vi "HFRR ADV v013 new software.vi"() -> ()   [LabVIEW 2025] (continued)
              n2046 = Add(x=w2266, y=0.0) -> (x+y=w2262:dbl)
            }
            n2047 = for {
              N: w2154 -> [_]
              tunnel: w2161 -> [w2209]
              tunnel: w2160 -> [w2208]
              tunnel: [w2198] -> w2114 mode=indexing
              tunnel: [w2197] -> w2107 mode=indexing
              tunnel: w2151 -> [_]
              tunnel: [w2186] -> w2112 mode=indexing
              tunnel: [w2191] -> w2109 mode=indexing
              tunnel: [w2187] -> w2099 mode=indexing
              tunnel: [w2182] -> w2074 mode=indexing
              tunnel: [w2178] -> w2055 mode=indexing
              tunnel: [w2173] -> w2015 mode=indexing
              (unwired) 1.0 ("x")
              (unwired) TRUE ("line mode (F)")
              n2048 = Read from Text File "Read File"(file (use dialog)=w2209, error in=w2208) -> (text=w2174:string)  [unwired: 2 in, 3 out]
              n2049 = local write "String 12"(w2174) -> ()
              n2050 = String Subset(string=w2174, offset (0)=85, length (rest)=9 ("length (rest)")) -> (substring=w2176:string)
              n2051 = String Subset(string=w2174, offset (0)=35, length (rest)=9 ("length (rest)")) -> (substring=w2199:string)
              n2052 = String Subset(string=w2174, offset (0)=55, length (rest)=9 ("length (rest)")) -> (substring=w2184:string)
              n2053 = String Subset(string=w2174, offset (0)=25, length (rest)=9 ("length (rest)")) -> (substring=w2180:string)
              n2054 = String Subset(string=w2174, offset (0)=45, length (rest)=9 ("length (rest)")) -> (substring=w2189:string)
              n2055 = String Subset(string=w2174, offset (0)=15, length (rest)=9 ("length (rest)")) -> (substring=w2205:string)
              n2056 = String Subset(string=w2174, offset (0)=0, length (rest)=14 ("length (rest)")) -> (substring=w2202:string)
              n2057 = String Subset(string=w2174, offset (0)=65, length (rest)=9 ("length (rest)")) -> (substring=w2192:string)
              n2058 = Fract/Exp String To Number(string=w2176) -> (number=w2173:dbl)  [unwired: 3 in, 1 out]
              n2059 = Fract/Exp String To Number(string=w2199) -> (number=w2197:dbl)  [unwired: 3 in, 1 out]
              n2060 = Fract/Exp String To Number(string=w2184) -> (number=w2182:dbl)  [unwired: 3 in, 1 out]
              n2061 = Fract/Exp String To Number(string=w2180) -> (number=w2178:dbl)  [unwired: 3 in, 1 out]
              n2062 = Fract/Exp String To Number(string=w2189) -> (number=w2187:dbl)  [unwired: 3 in, 1 out]
              n2063 = Fract/Exp String To Number(string=w2205) -> (number=w2186:dbl)  [unwired: 3 in, 1 out]
              n2064 = Fract/Exp String To Number(string=w2202) -> (number=w2198:dbl)  [unwired: 3 in, 1 out]
              n2065 = Fract/Exp String To Number(string=w2192) -> (number=w2195:dbl)  [unwired: 3 in, 1 out]
              n2066 = Add(x=w2195, y=0.0) -> (x+y=w2191:dbl)
            }
            n2067 = Delete From Array(array=w2057, index=0) -> (array with subset deleted=w2030:dbl[])  [unwired: 1 in, 1 out]
            n2068 = Delete From Array(array=w2120, index=0) -> (array with subset deleted=w2093:dbl[])  [unwired: 1 in, 1 out]
            n2069 = Delete From Array(array=w2100, index=0) -> (array with subset deleted=w2088:dbl[])  [unwired: 1 in, 1 out]
            n2070 = Delete From Array(array=w2118, index=0) -> (array with subset deleted=w2119:dbl[])  [unwired: 1 in, 1 out]
            n2071 = call-poly <vilib>:"Mean.vi"("X"=w2030) -> ("mean"=→"КОФ2 4":dbl)  [unwired: 1 out]
            n2072 = call-poly <vilib>:"Mean.vi"("X"=w2093) -> ("mean"=→"КОФ3":dbl)  [unwired: 1 out]
            n2073 = call-poly <vilib>:"Mean.vi"("X"=w2088) -> ("mean"=→"CP3":dbl)  [unwired: 1 out]
            n2074 = Delete From Array(array=w2082, index=0) -> (array with subset deleted=w2009:dbl[])  [unwired: 1 in, 1 out]
            n2075 = Delete From Array(array=w2021, index=0) -> (array with subset deleted=w2008:dbl[])  [unwired: 1 in, 1 out]
            n2076 = Delete From Array(array=w2061, index=0) -> (array with subset deleted=w2032:dbl[])  [unwired: 1 in, 1 out]
            n2077 = Delete From Array(array=w2139, index=0) -> (array with subset deleted=w2094:dbl[])  [unwired: 1 in, 1 out]
            n2078 = Delete From Array(array=w2105, index=0) -> (array with subset deleted=w2090:dbl[])  [unwired: 1 in, 1 out]
            "array w/ subset deleted" <- w2090
            n2079 = Delete From Array(array=w2136, index=0) -> (array with subset deleted=w2137:dbl[])  [unwired: 1 in, 1 out]
            n2080 = call-poly <vilib>:"Mean.vi"("X"=w2032) -> ("mean"=→"КОФ2 2":dbl)  [unwired: 1 out]
            n2081 = call-poly <vilib>:"Mean.vi"("X"=w2094) -> ("mean"=→"КОФ1":dbl)  [unwired: 1 out]
            n2082 = Bundle "Bundle"(w2009, w2008) -> (w2014:cluster{dbl[], dbl[]})  [unwired: 1 in]
            n2083 = Bundle "Bundle"(w2009, w2137) -> (w2001:cluster{dbl[], dbl[]})  [unwired: 1 in]
            n2084 = Delete From Array(array=w2016, index=0) -> (array with subset deleted=w2004:dbl[])  [unwired: 1 in, 1 out]
            n2085 = Delete From Array(array=w2017, index=0) -> (array with subset deleted=w2006:dbl[])  [unwired: 1 in, 1 out]
            n2086 = Delete From Array(array=w2127, index=0) -> (array with subset deleted=w2128:dbl[])  [unwired: 1 in, 1 out]
            n2087 = Delete From Array(array=w2015, index=0) -> (array with subset deleted=w2002:dbl[])  [unwired: 1 in, 1 out]
            n2088 = Delete From Array(array=w2109, index=0) -> (array with subset deleted=w2110:dbl[])  [unwired: 1 in, 1 out]
            n2089 = Delete From Array(array=w2134, index=0) -> (array with subset deleted=w2040:dbl[])  [unwired: 1 in, 1 out]
            n2090 = Delete From Array(array=w2080, index=0) -> (array with subset deleted=w2036:dbl[])  [unwired: 1 in, 1 out]
            n2091 = Delete From Array(array=w2116, index=0) -> (array with subset deleted=w2038:dbl[])  [unwired: 1 in, 1 out]
            n2092 = Delete From Array(array=w2076, index=0) -> (array with subset deleted=w2034:dbl[])  [unwired: 1 in, 1 out]
            n2093 = Delete From Array(array=w2125, index=0) -> (array with subset deleted=w2039:dbl[])  [unwired: 1 in, 1 out]
            n2094 = Delete From Array(array=w2078, index=0) -> (array with subset deleted=w2035:dbl[])  [unwired: 1 in, 1 out]
            n2095 = Delete From Array(array=w2059, index=0) -> (array with subset deleted=w2031:dbl[])  [unwired: 1 in, 1 out]
            n2096 = Delete From Array(array=w2103, index=0) -> (array with subset deleted=w2089:dbl[])  [unwired: 1 in, 1 out]
            n2097 = Delete From Array(array=w2130, index=0) -> (array with subset deleted=w2091:dbl[])  [unwired: 1 in, 1 out]
            n2098 = Delete From Array(array=w2107, index=0) -> (array with subset deleted=w2037:dbl[])  [unwired: 1 in, 1 out]
            n2099 = Delete From Array(array=w2074, index=0) -> (array with subset deleted=w2033:dbl[])  [unwired: 1 in, 1 out]
            n2100 = Delete From Array(array=w2055, index=0) -> (array with subset deleted=w2029:dbl[])  [unwired: 1 in, 1 out]
            n2101 = Delete From Array(array=w2099, index=0) -> (array with subset deleted=w2087:dbl[])  [unwired: 1 in, 1 out]
            n2102 = Delete From Array(array=w2112, index=0) -> (array with subset deleted=w2092:dbl[])  [unwired: 1 in, 1 out]
            n2103 = Delete From Array(array=w2122, index=0) -> (array with subset deleted=w2005:dbl[])  [unwired: 1 in, 1 out]
            n2104 = Delete From Array(array=w2132, index=0) -> (array with subset deleted=w2007:dbl[])  [unwired: 1 in, 1 out]
            n2105 = Delete From Array(array=w2114, index=0) -> (array with subset deleted=w2003:dbl[])  [unwired: 1 in, 1 out]
            n2106 = Bundle "Bundle"(w2009, w2040) -> (w2027:cluster{dbl[], dbl[]})  [unwired: 1 in]
            n2107 = Bundle "Bundle"(w2009, w2094) -> (w2028:cluster{dbl[], dbl[]})  [unwired: 1 in]
            n2108 = Bundle "Bundle"(w2040, w2036) -> (w2042:cluster{dbl[], dbl[]})  [unwired: 1 in]
            n2109 = Bundle "Bundle"(w2005, w2004) -> (w2012:cluster{dbl[], dbl[]})  [unwired: 1 in]
            n2110 = Bundle "Bundle"(w2038, w2034) -> (w2044:cluster{dbl[], dbl[]})  [unwired: 1 in]
            n2111 = Bundle "Bundle"(w2005, w2038) -> (w2148:cluster{dbl[], dbl[]})  [unwired: 1 in]
            n2112 = Bundle "Bundle"(w2005, w2034) -> (w2072:cluster{dbl[], dbl[]})  [unwired: 1 in]
            n2113 = Bundle "Bundle"(w2005, w2093) -> (w2158:cluster{dbl[], dbl[]})  [unwired: 1 in]
            n2114 = Bundle "Bundle"(w2005, w2088) -> (w2096:cluster{dbl[], dbl[]})  [unwired: 1 in]
            n2115 = Bundle "Bundle"(w2005, w2119) -> (w2143:cluster{dbl[], dbl[]})  [unwired: 1 in]
            n2116 = Bundle "Bundle"(w2039, w2035) -> (w2043:cluster{dbl[], dbl[]})  [unwired: 1 in]
            n2117 = Bundle "Bundle"(w2007, w2006) -> (w2013:cluster{dbl[], dbl[]})  [unwired: 1 in]
            n2118 = Bundle "Bundle"(w2007, w2039) -> (w2150:cluster{dbl[], dbl[]})  [unwired: 1 in]
            n2119 = Bundle "Bundle"(w2007, w2035) -> (w2073:cluster{dbl[], dbl[]})  [unwired: 1 in]
            n2120 = Bundle "Bundle"(w2007, w2089) -> (w2097:cluster{dbl[], dbl[]})  [unwired: 1 in]
            n2121 = Bundle "Bundle"(w2007, w2091) -> (w2159:cluster{dbl[], dbl[]})  [unwired: 1 in]
            n2122 = Bundle "Bundle"(w2007, w2128) -> (w2141:cluster{dbl[], dbl[]})  [unwired: 1 in]
            n2123 = Bundle "Bundle"(w2037, w2033) -> (w2045:cluster{dbl[], dbl[]})  [unwired: 1 in]
            n2124 = Bundle "Bundle"(w2003, w2002) -> (w2011:cluster{dbl[], dbl[]})  [unwired: 1 in]
            n2125 = Bundle "Bundle"(w2003, w2037) -> (w2149:cluster{dbl[], dbl[]})  [unwired: 1 in]
            n2126 = Bundle "Bundle"(w2003, w2033) -> (w2071:cluster{dbl[], dbl[]})  [unwired: 1 in]
            n2127 = Bundle "Bundle"(w2003, w2087) -> (w2095:cluster{dbl[], dbl[]})  [unwired: 1 in]
            n2128 = Bundle "Bundle"(w2003, w2092) -> (w2157:cluster{dbl[], dbl[]})  [unwired: 1 in]
            n2129 = Bundle "Bundle"(w2003, w2110) -> (w2142:cluster{dbl[], dbl[]})  [unwired: 1 in]
            n2130 = call-poly <vilib>:"Mean.vi"("X"=w2090) -> ("mean"=→"CP1":dbl)  [unwired: 1 out]
            n2131 = call-poly <vilib>:"Mean.vi"("X"=w2031) -> ("mean"=→"КОФ2 3":dbl)  [unwired: 1 out]
            n2132 = call-poly <vilib>:"Mean.vi"("X"=w2089) -> ("mean"=→"CP2":dbl)  [unwired: 1 out]
            n2133 = call-poly <vilib>:"Mean.vi"("X"=w2091) -> ("mean"=→"КОФ2":dbl)  [unwired: 1 out]
            n2134 = call-poly <vilib>:"Mean.vi"("X"=w2029) -> ("mean"=→"КОФ2 5":dbl)  [unwired: 1 out]
            n2135 = call-poly <vilib>:"Mean.vi"("X"=w2087) -> ("mean"=→"CP4":dbl)  [unwired: 1 out]
            n2136 = call-poly <vilib>:"Mean.vi"("X"=w2092) -> ("mean"=→"КОФ4":dbl)  [unwired: 1 out]
            n2137 = Bundle "Bundle"(w2009, w2036) -> (w2000:cluster{dbl[], dbl[]})  [unwired: 1 in]
            n2138 = Bundle "Bundle"(w2009, w2090) -> (w2023:cluster{dbl[], dbl[]})  [unwired: 1 in]
            n2139 = Build Array "Build Array"(w2000, w2023) -> (w2026:cluster{dbl[], dbl[]}[])
            "XY Graph 17" <- w2026
            n2140 = Build Array "Build Array"(w2014, w2013, w2012, w2011) -> (→"Frequency ( Hz )":cluster{dbl[], dbl[]}[])
            n2141 = Build Array "Build Array"(w2042, w2043, w2044, w2045) -> (→"Air Temp ( °C ) vs Humidity ( % RH )":cluster{dbl[], dbl[]}[])
            n2142 = Build Array "Build Array"(w2027, w2150, w2148, w2149) -> (→"Air Temperature  ( °C )":cluster{dbl[], dbl[]}[])
            n2143 = Build Array "Build Array"(w2000, w2073, w2072, w2071) -> (→"Humidity ( %RH )":cluster{dbl[], dbl[]}[])
            n2144 = Build Array "Build Array"(w2028, w2159, w2158, w2157) -> (→"Coefficient Of Friction":cluster{dbl[], dbl[]}[])
            n2145 = Build Array "Build Array"(w2023, w2097, w2096, w2095) -> (→"Sample Temperature ( °C )":cluster{dbl[], dbl[]}[])
            n2146 = Build Array "Build Array"(w2001, w2141, w2143, w2142) -> (→"XY Graph 13":cluster{dbl[], dbl[]}[])
            n2147 = Bundle "Bundle"(w2009, w2032) -> (w2054:cluster{dbl[], dbl[]})  [unwired: 1 in]
            n2148 = Bundle "Bundle"(w2005, w2030) -> (w2052:cluster{dbl[], dbl[]})  [unwired: 1 in]
            n2149 = Bundle "Bundle"(w2007, w2031) -> (w2053:cluster{dbl[], dbl[]})  [unwired: 1 in]
            n2150 = Bundle "Bundle"(w2003, w2029) -> (w2051:cluster{dbl[], dbl[]})  [unwired: 1 in]
            n2151 = Build Array "Build Array"(w2054, w2053, w2052, w2051) -> (→"Stroke ( mm )":cluster{dbl[], dbl[]}[])
            n2152 = local write "XY Graph 16"(w2026) -> ()
          }
          frame #2 {
          }
          frame #3 {
            n2153 = local write "Numeric 8"(0 ("Numeric 8")) -> ()
            n2154 = local write "Numeric 11"(0 ("Numeric 11")) -> ()
            n2155 = local write "Numeric 12"(0 ("Numeric 12")) -> ()
            n2156 = local write "Numeric 13"(0 ("Numeric 13")) -> ()
            n2157 = property on="OPEN" class="Bool (strict)"("Visible"=TRUE) -> ()  [unwired: 2 in, 2 out]
            n2158 = local read "String Control 2"() -> (w2326:string)
            n2159 = local read "String Control 4"() -> (w2325:string)
            n2160 = local read "String Control 6"() -> (w2324:string)
            n2161 = local read "String Control 8"() -> (w2323:string)
            n2162 = Match Pattern(string=w2326, regular expression="Samples / cycle :- ") -> (after substring=w2340:string)  [unwired: 1 in, 3 out]
            n2163 = Match Pattern(string=w2326, regular expression="Frequency :- ") -> (after substring=w2359:string)  [unwired: 1 in, 3 out]
            n2164 = Match Pattern(string=w2325, regular expression="Samples / cycle :- ") -> (after substring=w2336:string)  [unwired: 1 in, 3 out]
            n2165 = Match Pattern(string=w2325, regular expression="Frequency :- ") -> (after substring=w2354:string)  [unwired: 1 in, 3 out]
            n2166 = Match Pattern(string=w2324, regular expression="Samples / cycle :- ") -> (after substring=w2332:string)  [unwired: 1 in, 3 out]
            n2167 = Match Pattern(string=w2324, regular expression="Frequency :- ") -> (after substring=w2349:string)  [unwired: 1 in, 3 out]
            n2168 = Match Pattern(string=w2323, regular expression="Samples / cycle :- ") -> (after substring=w2328:string)  [unwired: 1 in, 3 out]
            n2169 = Match Pattern(string=w2323, regular expression="Frequency :- ") -> (after substring=w2344:string)  [unwired: 1 in, 3 out]
            n2170 = String Subset(string=w2340, length (rest)=6 ("length (rest)")) -> (substring=w2342:string)  [unwired: 1 in]
            n2171 = String Subset(string=w2359, length (rest)=9 ("length (rest)")) -> (substring=w2361:string)  [unwired: 1 in]
            n2172 = String Subset(string=w2336, length (rest)=6 ("length (rest)")) -> (substring=w2338:string)  [unwired: 1 in]
            n2173 = String Subset(string=w2354, length (rest)=9 ("length (rest)")) -> (substring=w2356:string)  [unwired: 1 in]
            n2174 = String Subset(string=w2332, length (rest)=6 ("length (rest)")) -> (substring=w2334:string)  [unwired: 1 in]
            n2175 = String Subset(string=w2349, length (rest)=9 ("length (rest)")) -> (substring=w2351:string)  [unwired: 1 in]
            n2176 = String Subset(string=w2328, length (rest)=6 ("length (rest)")) -> (substring=w2330:string)  [unwired: 1 in]
            n2177 = String Subset(string=w2344, length (rest)=9 ("length (rest)")) -> (substring=w2346:string)  [unwired: 1 in]
            n2178 = Fract/Exp String To Number(string=w2342) -> (number=w2322:dbl)  [unwired: 3 in, 1 out]
            n2179 = Fract/Exp String To Number(string=w2361) -> (number=w2362:dbl)  [unwired: 3 in, 1 out]
            n2180 = Fract/Exp String To Number(string=w2338) -> (number=w2321:dbl)  [unwired: 3 in, 1 out]
            n2181 = Fract/Exp String To Number(string=w2356) -> (number=w2357:dbl)  [unwired: 3 in, 1 out]
            n2182 = Fract/Exp String To Number(string=w2334) -> (number=w2320:dbl)  [unwired: 3 in, 1 out]
            n2183 = Fract/Exp String To Number(string=w2351) -> (number=w2352:dbl)  [unwired: 3 in, 1 out]
            n2184 = Fract/Exp String To Number(string=w2330) -> (number=w2319:dbl)  [unwired: 3 in, 1 out]
            n2185 = Fract/Exp String To Number(string=w2346) -> (number=w2347:dbl)  [unwired: 3 in, 1 out]
            n2186 = local write "sample1"(w2322) -> ()
            n2187 = local write "freq1"(w2362) -> ()
            n2188 = local write "sample2"(w2321) -> ()
            n2189 = local write "freq2"(w2357) -> ()
            n2190 = local write "sample3"(w2320) -> ()
            n2191 = local write "freq3"(w2352) -> ()
            n2192 = local write "sample4"(w2319) -> ()
            n2193 = local write "freq 4"(w2347) -> ()
          }
        }
      }
    }
    n2194 = case shown="True" w1811 {
      selector: w1811 -> [_ w1939]
      frame False {
      }
      frame True {
        n2195 = Not(x=w1939) -> (.not. x?=w1935:bool)
        n2196 = local write "service 3"(w1935) -> ()
        n2197 = local write "OPEN 6"(w1935) -> ()
        n2198 = call <vilib>:"System Exec.vi"("wait until completion? (T)"=TRUE, "command line"="C:\\LAB-IQ\\Scar View.exe") -> ("error out"=→"error out 5":errorcluster)  [unwired: 6 in, 3 out]
      }
    }
    n2199 = case shown="\"Acquire\", Default" w1822 {
      frame "Acquire", Default {
        w2835 = 0.2 ("y")
        w2840 = 1.0 ("y")
        w2841 = 0.8 ("y")
        # "Elapsed time\ncof\nstroke\nAir temp\nTemp\nHumidity"
        n2200 = disable-structure shown="Disabled" {
          frame Disabled {
            n2201 = local read "Flag"() -> (w2858:dbl)
            n2202 = local read "RUN"() -> (w2855:bool)
            n2203 = Not(x=w2855) -> (.not. x?=w2854:bool)
            n2204 = Equal?(x=w2858, y=10.0) -> (x = y?=w2856:bool)
            n2205 = And(x=w2856, y=w2854) -> (x .and. y?=w2853:bool)
            n2206 = case shown="True" w2853 {
              frame False {
              }
              frame True {
                w2859 = FALSE ("Heater Button")
                n2207 = local write "Humidity"(w2859) -> ()
                n2208 = local write "Heater Button"(w2859) -> ()
              }
            }
          }
          frame Enabled {
          }
        }
        n2209 = disable-structure shown="Disabled" {
          frame Disabled {
            n2210 = case shown="True" {
              selector: _ -> [_ _]
              frame False {
              }
              frame True {
                w2950 = TRUE ("Heater")
                n2211 = local write "Humidity"(w2950) -> ()
                n2212 = local write "Heater Button"(w2950) -> ()
                n2213 = local read "TEST STANDARD"() -> (w2953:T3)
                n2214 = local read "TEST STANDARD"() -> (w2948:T3)
                n2215 = Equal?(x=w2953, y=enum16{"ASTM D6079", "ISO 12156", "Custom"}."ISO 12156" ("Test Standard")) -> (x = y?=w2951:bool)
                n2216 = Equal?(x=w2948, y=enum16{"ASTM D6079", "ISO 12156", "Custom"}."ASTM D6079" ("Test Standard")) -> (x = y?=w2947:bool)
                n2217 = case shown="True" w2951 {
                  frame False {
                  }
                  frame True {
                    n2218 = local write "Heater"(TRUE ("Heater")) -> ()
                    n2219 = local write "airtempflg"(FALSE ("airtempflg")) -> ()
                  }
                }
                n2220 = case shown="True" w2947 {
                  frame False {
                  }
                  frame True {
                    n2221 = local write "Heater"(FALSE ("Heater")) -> ()
                    n2222 = local write "airtempflg"(TRUE ("airtempflg")) -> ()
                  }
                }
              }
            }
          }
          frame Enabled {
          }
        }
        n2223 = stacked-sequence {
          frame #0 {
            n2224 = case shown="True" "RST FF" {
              frame False {
              }
              frame True {
                w3016 = 0.0 ("X Scale.Range:Maximum")
                n2225 = property on="Frictional Force ( N )" class="WFChart (strict)"("XScale.Maximum"=600.0 ("X Scale.Range:Maximum"), "XScale.Minimum"=w3016, "YScale.Maximum"=10.0 ("Y Scale.Range:Maximum"), "YScale.Minimum"=w3016) -> ()  [unwired: 2 in, 2 out]
              }
            }
          }
          frame #1 {
            n2226 = case shown="True" "RST TEMP" {
              frame False {
              }
              frame True {
                n2227 = property on="Temperature ( Deg C )" class="WFChart (strict)"("XScale.Minimum"=0.0 ("X Scale.Range:Minimum"), "XScale.Maximum"=600.0 ("X Scale.Range:Maximum"), "YScale.Minimum"=0.0 ("Y Scale.Range:Minimum"), "YScale.Maximum"=100.0 ("Y Scale.Range:Maximum")) -> ()  [unwired: 2 in, 2 out]
              }
            }
          }
          frame #2 {
            n2228 = case shown="True" "RSTCOF" {
              frame False {
              }
              frame True {
                n2229 = property on="Coefficient of Friction" class="WFChart (strict)"("XScale.Minimum"=0.0 ("X Scale.Range:Minimum"), "XScale.Maximum"=600.0 ("X Scale.Range:Maximum"), "YScale.Maximum"=1.0 ("X Scale.Range:Minimum"), "YScale.Minimum"=0.0 ("X Scale.Range:Minimum")) -> ()  [unwired: 2 in, 2 out]
              }
            }
          }
          frame #3 {
            n2230 = case shown="True" "RSTCOF 2" {
              frame False {
              }
              frame True {
                (unwired) 100.0 ("Y Scale.Range:Maximum")
                (unwired) 0.0 ("Y Scale.Range:Minimum")
                (unwired) 600.0 ("X Scale.Range:Maximum")
                (unwired) 0.0 ("X Scale.Range:Minimum")
              }
            }
          }
          frame #4 {
            n2231 = case shown="True" "RSTCOF 3" {
              frame False {
              }
              frame True {
                n2232 = property on="Electrical Contact Resistance ( % )" class="WFChart (strict)"("XScale.Minimum"=0.0 ("X Scale.Range:Minimum"), "XScale.Maximum"=600.0 ("X Scale.Range:Maximum"), "YScale.Minimum"=0.0 ("Y Scale.Range:Minimum"), "YScale.Maximum"=100.0 ("Y Scale.Range:Maximum")) -> ()  [unwired: 2 in, 2 out]
              }
            }
          }
        }
        n2233 = disable-structure shown="Disabled" {
          frame Disabled {
            n2234 = case shown="True" {
              selector: _ -> [_ _]
              frame False {
              }
              frame True {
                n2235 = local read "zflag 2"() -> (w2917:dbl)
                n2236 = local read "yflag"() -> (w2919:dbl)
                n2237 = Equal?(x=w2919, y=2.0 ("tflag")) -> (x = y?=w2921:bool)
                n2238 = Equal?(x=w2917, y=3.0 ("tflag")) -> (x = y?=w2920:bool)
                n2239 = And(x=w2921, y=w2920) -> (x .and. y?=w2915:bool)
                n2240 = case shown="True" w2915 {
                  frame False {
                  }
                  frame True {
                    w2946 = 0.0 ("zflag")
                    n2241 = local write "zflag"(w2946) -> ()
                    n2242 = local write "zflag 2"(w2946) -> ()
                    n2243 = Delete(path (use dialog)=path "C:/LAB-IQ-NXT/WO 2449 TT.sig" ("file path (dialog if empty)")) -> (deleted path=w2945:path)  [unwired: 4 in, 2 out]
                    n2244 = Delete(path (use dialog)=path "C:/LAB-IQ-NXT/WO 2449 TRH.sig" ("file path (dialog if empty)")) -> (deleted path=w2940:path)  [unwired: 4 in, 2 out]
                    n2245 = local read "SEN.RUN HRS"() -> (w2932:dbl)
                    n2246 = local read "SENSOR TIME"() -> (w2930:dbl)
                    n2247 = call <vilib>:"compatOverwrite.vi"("overwrite (F)"=TRUE) -> ("overwrite?"=w2922:T29)
                    n2248 = call <vilib>:"compatOverwrite.vi"("overwrite (F)"=TRUE) -> ("overwrite?"=w2926:T29)
                    n2249 = local read "Total No. of Tests"() -> (w2933:dbl)
                    n2250 = Add(x=w2930, y=w2932) -> (x+y=w2931:dbl)
                    "SEN.RUN HRS" <- w2931
                    n2251 = Open/Create/Replace File(file path (use dialog)=w2945, operation (0:open)=w2922) -> (refnum out=w2923:refnum<file>, error out=w2924:errorcluster)  [unwired: 4 in, 1 out]
                    n2252 = Open/Create/Replace File(file path (use dialog)=w2940, operation (0:open)=w2926) -> (refnum out=w2927:refnum<file>, error out=w2928:errorcluster)  [unwired: 4 in, 1 out]
                    n2253 = Deny Access(4:w2924, 6:T27."deny none" ("deny mode (2)"), 7:w2923) -> (3:w2944:refnum<file>)  [unwired: 1 out]
                    n2254 = Deny Access(4:w2928, 6:T27."deny none" ("deny mode (2)"), 7:w2927) -> (3:w2936:refnum<file>)  [unwired: 1 out]
                    n2255 = Number To Decimal String(number=w2933) -> (decimal integer string=w2941:string)  [unwired: 1 in]
                    n2256 = Number To Decimal String(number=w2931) -> (decimal integer string=w2937:string)  [unwired: 1 in]
                    n2257 = Write to Binary File(file (use dialog)=w2944, data=w2941, 5:FALSE ("prepend array or string size? (T)")) -> ()  [unwired: 3 in, 3 out]
                    n2258 = Write to Binary File(file (use dialog)=w2936, data=w2937, 5:FALSE ("prepend array or string size? (T)")) -> ()  [unwired: 3 in, 3 out]
                  }
                }
              }
            }
          }
          frame Enabled {
          }
        }
        n2259 = local read "RUN"() -> (w2844:bool)
        n2260 = local read "run replace"() -> (w2848:bool)
        n2261 = local read "run replace"() -> (w2847:bool)
        n2262 = case shown="True" w2844 {
          frame False {
            n2263 = local write "run replace"(FALSE ("run replace")) -> ()
          }
          frame True {
            "run replace" <- TRUE ("run replace")
          }
        }
        n2264 = local read "RUN"() -> (w2852:bool)
        n2265 = local read "Set Temp"() -> (w2814:dbl)
        n2266 = local read "SetTemp"() -> (w2816:dbl)
        n2267 = case shown="False" w2852 {
          tunnel: [FALSE ("TEST RUNNING") TRUE ("TEST RUNNING")] -> w2851
          frame False {
            w3035 = 0.0 ("Flag")
            n2268 = local write "Elapsed time"(0.0 ("elapsedtime")) -> ()
            n2269 = local write "Time Remaining"(w3035) -> ()
            n2270 = local write "Flag"(w3035) -> ()
            n2271 = local write "Remaining Time"(w3035) -> ()
          }
          frame True {
            n2272 = local write "Flag"(10.0 ("Flag")) -> ()
          }
        }
        n2273 = case shown="False" w2848 {
          frame False {
            n2274 = local read "zflag"() -> (→"zflag 2":dbl)
            n2275 = local write "yflag"(2.0 ("tflag")) -> ()
            n2276 = local write "FLAG 4"(0.0 ("FLAG")) -> ()
          }
          frame True {
            n2277 = local write "yflag"(1.0 ("tflag")) -> ()
            n2278 = local write "zflag"(3.0 ("zflag")) -> ()
          }
        }
        n2279 = local read "acq 2"() -> (w2846:bool)
        n2280 = local read "AIR TEMP"() -> (w2809:dbl)
        n2281 = local read "Amb temp"() -> (w2813:dbl)
        n2282 = case shown="True" "Save & Continue" {
          frame False {
          }
          frame True {
            "acq 2" <- TRUE ("acq 2")
          }
        }
        n2283 = local read "Set Rh"() -> (w2815:dbl)
        n2284 = Add(x=w2816, y=w2841) -> (x+y=w2842:dbl)
        n2285 = Subtract(x=w2816, y=w2841) -> (x-y=w2843:dbl)
        n2286 = Add(x=w2814, y=w2835) -> (x+y=w2836:dbl)
        n2287 = Subtract(x=w2814, y=w2835) -> (x-y=w2837:dbl)
        n2288 = And(x=w2846, y=w2847) -> (x .and. y?=w2845:bool)
        n2289 = Greater Or Equal?(x=w2809, y=15.0) -> (x >= y?=w2810:bool)
        "powstat" <- w2810
        n2290 = local read "Humidity ( %RH )"() -> (w2812:dbl)
        n2291 = case shown="True" "Save & Continue" {
          frame False {
          }
          frame True {
            n2292 = while {
              tunnel: "0123456789abcdefghijklmnopqrstuvwxyzABCDEFGHIJKLMNOPQRSTUVWXYZ" ("string 2") -> [w3006]
              shift-right: [w3004] -> w2999
              shift-left: "" -> [w3003]
              i -> [w3013]
              stop <- w3012 stop-if-true
              n2293 = Random Number (0-1)() -> (number: 0 to 1=w3007:dbl)
              n2294 = Multiply(x=w3007, y=62.0) -> (x*y=w3009:dbl)
              n2295 = Decrement(x="Length") -> (x-1=w3002:i16)
              n2296 = To Word Integer(number=w3009) -> (16bit integer=w3010:i16)
              n2297 = String Subset(string=w3006, offset (0)=w3010, length (rest)=1 ("length (rest)")) -> (substring=w3005:string)
              n2298 = Greater Or Equal?(x=w3013, y=w3002) -> (x >= y?=w3012:bool)
              n2299 = Concatenate Strings(w3005, w3003) -> (w3004:string)
            }
            n2300 = local write "UUID"(w2999) -> ()
          }
        }
        n2301 = In Range and Coerce(upper limit=w2842, x=w2813, lower limit=w2843) -> (In Range?=w2832:bool)  [unwired: 1 out]
        n2302 = Add(x=w2815, y=w2840) -> (x+y=w2839:dbl)
        n2303 = Subtract(x=w2815, y=w2840) -> (x-y=w2838:dbl)
        n2304 = local read "TEMP"() -> (w2811:dbl)
        n2305 = case shown="True" "Save & Continue" {
          frame False {
          }
          frame True {
            n2306 = local read "Operator ID"() -> (w3330:string)
            n2307 = local read "FILE"() -> (w3336:string)
            n2308 = String Length(string=w3336) -> (length=w3334:i32)
            n2309 = String Length(string=w3330) -> (length=w3331:i32)
            n2310 = Greater?(x=w3334, y=0) -> (0:w3333:bool)
            n2311 = Greater?(x=w3331, y=0) -> (0:w3329:bool)
            n2312 = And(x=w3333, y=w3329) -> (x .and. y?=w3328:bool)
            n2313 = case shown="True" w3328 {
              frame False {
                n2314 = stacked-sequence {
                  frame #0 {
                    n2315 = One Button Dialog(message="Please Enter a File Name and Operator ID to save data !", button name ("OK")="Ok") -> ()  [unwired: 1 out]
                  }
                  frame #1 {
                    n2316 = local write "Save & Continue"(FALSE ("OK Button")) -> ()
                  }
                }
                n2317 = local write "Save & Continue"(FALSE ("OK Button")) -> ()
              }
              frame True {
                n2318 = stacked-sequence {
                  frame #0 {
                    n2319 = local read "FILE"() -> (w3342:string)
                    n2320 = call "file check.vi"("file name in"=w3342) -> ("file name out"=w3341:string)  [unwired: 9 in, 1 out]
                    n2321 = call <vilib>:"Application Directory.vi"() -> ("Application Directory"=w3352:path)
                    n2322 = Build Path(base path=w3352, name or relative path="data") -> (appended path=w3351:path)
                    n2323 = call <vilib>:"Trim Whitespace.vi"("string"=w3341) -> ("trimmed string"=w3349:string)  [unwired: 1 in]
                    n2324 = call <vilib>:"Trim Whitespace.vi"("string"=w3341) -> ("trimmed string"=w3350:string)  [unwired: 1 in]
                    n2325 = List Folder(path=w3351) -> (folder names=w3347:string[])  [unwired: 3 in, 3 out]
                    n2326 = Match Pattern(string=w3349, regular expression="_(") -> (before substring=w3346:string)  [unwired: 1 in, 3 out]
                    n2327 = for {
                      tunnel: w3347 -> [w3361] mode=indexing
                      tunnel: w3346 -> [w3359]
                      shift-right: [w3357] -> w3344
                      shift-left: bool[] [] -> [w3358]
                      n2328 = Match Pattern(string=w3361, regular expression="_(") -> (before substring=w3360:string)  [unwired: 1 in, 3 out]
                      n2329 = Equal?(x=w3360, y=w3359) -> (x = y?=w3356:bool)
                      n2330 = case shown="True" w3356 {
                        tunnel: w3356 -> [_ w3364]
                        tunnel: w3358 -> [w3363 w3366]
                        tunnel: [w3363 w3365] -> w3357
                        frame False {
                        }
                        frame True {
                          n2331 = Insert Into Array(array=w3366, new element=w3364) -> (w3365:bool[])  [unwired: 1 in]
                        }
                      }
                    }
                    n2332 = Equal?(x=w3347, y=w3346) -> (x = y?=w3355:bool[])
                    n2333 = Or Array Elements(Boolean array=w3355) -> (logical OR=w3354:bool)
                    n2334 = Array Size(array=w3344) -> (size(s)=w3343:i32)
                    n2335 = case shown="True" w3354 {
                      tunnel: w3350 -> [_ w3374]
                      tunnel: w3343 -> [_ w3367]
                      frame False {
                      }
                      frame True {
                        n2336 = Number To Decimal String(number=w3367) -> (decimal integer string=w3370:string)  [unwired: 1 in]
                        n2337 = Search/Split String(string=w3374, search string/char (-)="_(" ("regular expression")) -> (substring before match=w3372:string)  [unwired: 1 in, 2 out]
                        n2338 = Concatenate Strings(w3372, "_(" ("regular expression"), w3370, ")" ("regular expression")) -> (w3368:string)
                        n2339 = local write "FILE"(w3368) -> ()
                      }
                    }
                  }
                  frame #1 {
                    w3376 = 0.0
                    w3389 = cluster{"y":dbl, dbl, "y":dbl}[] [] ("History Data")
                    w3390 = FALSE ("Heater Button")
                    (unwired) ")!" ("string")
                    (unwired) ")" ("string")
                    w3388 = dbl[] [] ("History Data")
                    w3394 = "\r"
                    # "C:\\WinDucom\\Data\\"
                    # "C:\\LAB-IQ-NXT\\data"
                    n2340 = local write "Humidity ( %RH )"(w3376) -> ()
                    n2341 = local write "Frequency ( Hz )"(w3376) -> ()
                    n2342 = local write "Stroke 3"(w3376) -> ()
                    n2343 = local write "speedop"(0.0 ("PIDclk 2")) -> ()
                    n2344 = local write "Set Temp 2"(65.0 ("Set Temp 2")) -> ()
                    n2345 = local write "AIR TEMP"(w3376) -> ()
                    n2346 = local write "clk"(0.0 ("clk")) -> ()
                    n2347 = local write "Stroke 4"(w3376) -> ()
                    n2348 = local write "COF 2"(w3376) -> ()
                    n2349 = local write "TEMP"(w3376) -> ()
                    n2350 = local write "ecr 3"(w3376) -> ()
                    n2351 = local write "FF 3"(w3376) -> ()
                    n2352 = local write "FF 2"(w3376) -> ()
                    n2353 = property on="Humidity ( %RH )" class="WFChart (strict)"("History Data"=w3388) -> ()  [unwired: 2 in, 2 out]
                    n2354 = property on="Coefficient of Friction" class="WFChart (strict)"("History Data"=w3388) -> ()  [unwired: 2 in, 2 out]
                    n2355 = property on="Coefficient of Friction" class="WFChart (strict)"("History Data"=w3388) -> ()  [unwired: 2 in, 2 out]
                    n2356 = property on="Frictional Force ( N )" class="WFChart (strict)"("History Data"=w3388) -> ()  [unwired: 2 in, 2 out]
                    n2357 = property on="Electrical Contact Resistance ( % )" class="WFChart (strict)"("History Data"=w3388) -> ()  [unwired: 2 in, 2 out]
                    n2358 = property on="Electrical Contact Resistance ( % )" class="WFChart (strict)"("History Data"=w3388) -> ()  [unwired: 2 in, 2 out]
                    n2359 = property on="Temperature ( Deg C )" class="WFChart (strict)"("History Data"=w3388) -> ()  [unwired: 2 in, 2 out]
                    n2360 = property on="Frictional Force ( N )" class="WFChart (strict)"("History Data"=w3388) -> ()  [unwired: 2 in, 2 out]
                    n2361 = property on="Coefficient of Friction" class="WFChart (strict)"("History Data"=w3388) -> ()  [unwired: 2 in, 2 out]
                    n2362 = property on="Frictional Force ( N )" class="WFChart (strict)"("History Data"=w3388) -> ()  [unwired: 2 in, 2 out]
                    n2363 = property on="Electrical Contact Resistance ( % )" class="WFChart (strict)"("History Data"=w3388) -> ()  [unwired: 2 in, 2 out]
                    n2364 = property on="Temperature ( Deg C )" class="WFChart (strict)"("History Data"=w3388) -> ()  [unwired: 2 in, 2 out]
                    n2365 = property on="Humidity ( %RH )" class="WFChart (strict)"("History Data"=w3388) -> ()  [unwired: 2 in, 2 out]
                    n2366 = property on="Stroke ( mm )" class="WFChart (strict)"("History Data"=w3389) -> ()  [unwired: 2 in, 2 out]
                    n2367 = property on="Stroke ( mm )" class="WFChart (strict)"("History Data"=w3389) -> ()  [unwired: 2 in, 2 out]
                    n2368 = local write "Humidity"(w3390) -> ()
                    n2369 = local write "Heater Button"(w3390) -> ()
                    n2370 = local read "FILE"() -> (w3384:string)
                    n2371 = disable-structure shown="Enabled" {
                      disable-tunnel: [w3429 _] -> w3375
                      frame Enabled {
                        n2372 = local read "NORMAL LOAD"() -> (w3429:dbl)
                      }
                      frame Disabled {
                      }
                    }
                    n2373 = call "file check.vi"("file name in"=w3384) -> ("error out"=w3387:errorcluster, "file name out"=w3381:string)  [unwired: 9 in]
                    n2374 = call "FILE PATH CREATION.vi"("error in"=w3387, "FILE NAME :"=w3381) -> ("FILE OUT"=w3380:path)  [unwired: 8 in, 1 out]
                    n2375 = Concatenate Strings(w3381, ".dgf" ("Substring")) -> (w3386:string)
                    n2376 = Concatenate Strings(w3381, ".duf" ("Substring")) -> (w3382:string)
                    n2377 = Multiply(x=w3375, y=1.0) -> (x*y=w3408:dbl)
                    n2378 = Build Path(base path=w3380, name or relative path=w3386) -> (appended path=w3379:path)
                    n2379 = Build Path(base path=w3380, name or relative path=w3382) -> (appended path=w3378:path)
                    n2380 = Number To Fractional String(number=w3408, width (-)=i16 5, precision (6)=i16 2) -> (F-format string=w3416:string)  [unwired: 1 in]
                    n2381 = local read "Fuel Discription :"() -> (w3404:string)
                    n2382 = local read "Batch Ref Num :"() -> (w3392:string)
                    n2383 = Get Date/Time String(date format (0)=enum16{"short", "long", "abbreviated"}."short") -> (date string=w3427:string, time string=w3424:string)  [unwired: 2 in]
                    n2384 = local read "Remarks :"() -> (w3403:string)
                    n2385 = Concatenate Strings("Load :- " ("Substring"), w3416, " grams ," ("Substring")) -> (w3415:string)
                    n2386 = local read "String 41"() -> (w3395:string)
                    n2387 = Concatenate Strings(w3404) -> (w3405:string)
                    n2388 = Concatenate Strings(w3392) -> (w3391:string)
                    n2389 = Concatenate Strings("tested by") -> (w3399:string)
                    n2390 = Concatenate Strings("(" ("Substring"), w3427, ")" ("Substring"), w3424) -> (w3397:string)
                    "concatenated string" <- w3397
                    n2391 = Concatenate Strings(w3403, "," ("string")) -> (w3402:string)
                    n2392 = Concatenate Strings("  TIME;      COF;       STROKE;     AIR TEMP;  TEMP;  HUMIDITY;  ECR; PID-OUT; FREQUENCY" ("Substring"), "\r") -> (w3411:string)
                    n2393 = Concatenate Strings(w3395, w3394, "Fuel Discription :-" ("Substring"), w3405, w3394, w3415, w3394, "Batch Ref Num :-" ("Substring"), w3391, w3394, " Remarks :- " ("Substring"), w3402, w3394, " Date :- " ("Substring"), w3397, w3394, "Tested By :-" ("Substring"), w3399) -> (w3409:string)
                    "REMARKS" <- w3409
                    n2394 = call <vilib>:"Write Characters To File.vi"("append to file? (new file:F)"=FALSE, "character string"=w3411, "file path (dialog if empty)"=w3379) -> ()  [unwired: 2 in, 1 out]
                    n2395 = call <vilib>:"Write Characters To File.vi"("append to file? (new file:F)"=FALSE, "character string"=w3409, "file path (dialog if empty)"=w3378) -> ()  [unwired: 2 in, 1 out]
                  }
                  frame #2 {
                    n2396 = local write "Cycles elapsed"(0 ("Cycles elapsed")) -> ()
                    n2397 = local write "cyclecount"(0 ("cyclecount")) -> ()
                    n2398 = local write "Save & Continue"(FALSE ("OK")) -> ()
                    n2399 = local write "autostrtflg"(TRUE ("autostrtflg")) -> ()
                    n2400 = local write "Save"(FALSE ("Save")) -> ()
                    n2401 = Get Date/Time In Seconds() -> (seconds since 1Jan1904=w3434:timestamp)
                    n2402 = To Double Precision Float(number=w3434) -> (double precision float=w3433:dbl)
                    n2403 = local write "acq timer"(w3433) -> ()
                    n2404 = One Button Dialog(message="Please ensure sample is mounted properly and machine is ready in all aspects for testing !", button name ("OK")="Ok") -> ()  [unwired: 1 out]
                  }
                  frame #3 {
                    n2405 = stacked-sequence {
                      frame #0 {
                        n2406 = local write "Main Dashboard Buttons"(T1."Dashboard" ("Main Dashboard Buttons")) -> ()
                        n2407 = local write "Main Tab"(T2."Acquire" ("Main Tab")) -> ()
                      }
                      frame #1 {
                        n2408 = local write "EVENT LOG"("" ("EVENT LOG")) -> ()
                      }
                      frame #2 {
                        n2409 = Wait (ms)(milliseconds to wait=u32 50) -> ()  [unwired: 1 out]
                      }
                      frame #3 {
                        n2410 = disable-structure shown="Disabled" {
                          frame Disabled {
                            n2411 = local read "EVENT LOG"() -> (w3446:string)
                            n2412 = call "Event Log.vi"("Content"="Test Details", "EVENT LOG"=w3446) -> ("EVENT LOG"=w3445:string)  [unwired: 8 in, 1 out]
                            n2413 = local write "EVENT LOG"(w3445) -> ()
                          }
                          frame Enabled {
                          }
                        }
                      }
                      frame #4 {
                        n2414 = Wait (ms)(milliseconds to wait=u32 50) -> ()  [unwired: 1 out]
                      }
                      frame #5 {
                        n2415 = local read "FILE"() -> (w3448:string)
                        n2416 = Concatenate Strings("File Name :" ("Content"), w3448) -> (w3449:string)
                        n2417 = local read "EVENT LOG"() -> (w3452:string)
                        n2418 = call "Event Log.vi"("Content"=w3449, "EVENT LOG"=w3452) -> ("EVENT LOG"=w3451:string)  [unwired: 8 in, 1 out]
                        n2419 = local write "EVENT LOG"(w3451) -> ()
                      }
                      frame #6 {
                        n2420 = Wait (ms)(milliseconds to wait=u32 50) -> ()  [unwired: 1 out]
                      }
                      frame #7 {
                        n2421 = local read "Batch Ref Num :"() -> (w3454:string)
                        n2422 = Concatenate Strings("Batch Ref No :" ("Content"), w3454) -> (w3455:string)
                        n2423 = local read "EVENT LOG"() -> (w3458:string)
                        n2424 = call "Event Log.vi"("Content"=w3455, "EVENT LOG"=w3458) -> ("EVENT LOG"=w3457:string)  [unwired: 8 in, 1 out]
                        n2425 = local write "EVENT LOG"(w3457) -> ()
                      }
                      frame #8 {
                        n2426 = Wait (ms)(milliseconds to wait=u32 50) -> ()  [unwired: 1 out]
                      }
                      frame #9 {
                        n2427 = local read "tested by"() -> (w3460:string)
                        n2428 = Concatenate Strings("Tested By :" ("Content"), w3460) -> (w3461:string)
                        n2429 = local read "EVENT LOG"() -> (w3464:string)
                        n2430 = call "Event Log.vi"("Content"=w3461, "EVENT LOG"=w3464) -> ("EVENT LOG"=w3463:string)  [unwired: 8 in, 1 out]
                        n2431 = local write "EVENT LOG"(w3463) -> ()
                      }
                      frame #10 {
                        n2432 = Wait (ms)(milliseconds to wait=u32 50) -> ()  [unwired: 1 out]
                      }
                      frame #11 {
                        n2433 = local read "TEST STANDARD"() -> (w3467:T3)
                        n2434 = case shown="\"ASTM D6079\", Default" w3467 {
                          tunnel: ["ASTM D6079" "ISO 12156" "CEC F-096-A-06" "Custom"] -> w3466
                          frame "ASTM D6079", Default {
                          }
                          frame "ISO 12156" {
                          }
                          frame "CEC F-096-A-06" {
                          }
                          frame "Custom" {
                          }
                        }
                        n2435 = Concatenate Strings("Test Standard :" ("Content"), w3466) -> (w3468:string)
                        n2436 = local read "EVENT LOG"() -> (w3471:string)
                        n2437 = call "Event Log.vi"("Content"=w3468, "EVENT LOG"=w3471) -> ("EVENT LOG"=w3470:string)  [unwired: 8 in, 1 out]
                        n2438 = local write "EVENT LOG"(w3470) -> ()
                      }
                      frame #12 {
                        n2439 = Wait (ms)(milliseconds to wait=u32 50) -> ()  [unwired: 1 out]
                      }
                      frame #13 {
                        n2440 = local read "Fuel Discription :"() -> (w3477:string)
                        n2441 = Concatenate Strings("Fuel Description :" ("Content"), w3477) -> (w3478:string)
                        n2442 = local read "EVENT LOG"() -> (w3481:string)
                        n2443 = call "Event Log.vi"("Content"=w3478, "EVENT LOG"=w3481) -> ("EVENT LOG"=w3480:string)  [unwired: 8 in, 1 out]
                        n2444 = local write "EVENT LOG"(w3480) -> ()
                      }
                      frame #14 {
                        n2445 = Wait (ms)(milliseconds to wait=u32 50) -> ()  [unwired: 1 out]
                      }
                      frame #15 {
                        n2446 = local read "Remarks :"() -> (w3483:string)
                        n2447 = Concatenate Strings("Remarks :" ("Content"), w3483) -> (w3484:string)
                        n2448 = local read "EVENT LOG"() -> (w3487:string)
                        n2449 = call "Event Log.vi"("Content"=w3484, "EVENT LOG"=w3487) -> ("EVENT LOG"=w3486:string)  [unwired: 8 in, 1 out]
                        n2450 = local write "EVENT LOG"(w3486) -> ()
                      }
                      frame #16 {
                        n2451 = Wait (ms)(milliseconds to wait=u32 50) -> ()  [unwired: 1 out]
                      }
                      frame #17 {
                        n2452 = local read "Operator ID"() -> (w3489:string)
                        n2453 = Concatenate Strings("Operator ID :" ("Content"), w3489) -> (w3491:string)
                        n2454 = local read "EVENT LOG"() -> (w3493:string)
                        n2455 = call "Event Log.vi"("Content"=w3491, "EVENT LOG"=w3493) -> ("EVENT LOG"=w3492:string)  [unwired: 8 in, 1 out]
                        n2456 = local write "EVENT LOG"(w3492) -> ()
                      }
                      frame #18 {
                        n2457 = Wait (ms)(milliseconds to wait=u32 50) -> ()  [unwired: 1 out]
                      }
                      frame #19 {
                        n2458 = disable-structure shown="Disabled" {
                          frame Disabled {
                            n2459 = local read "EVENT LOG"() -> (w3497:string)
                            n2460 = call "Event Log.vi"("Content"="Test Parameter", "EVENT LOG"=w3497) -> ("EVENT LOG"=w3496:string)  [unwired: 8 in, 1 out]
                            n2461 = local write "EVENT LOG"(w3496) -> ()
                          }
                          frame Enabled {
                          }
                        }
                      }
                      frame #20 {
                        n2462 = Wait (ms)(milliseconds to wait=u32 50) -> ()  [unwired: 1 out]
                      }
                      frame #21 {
                        n2463 = local read "Set Hz"() -> (w3501:dbl)
                        n2464 = Number To Fractional String(number=w3501, precision (6)=i16 2) -> (F-format string=w3500:string)  [unwired: 2 in]
                        n2465 = Concatenate Strings("Set Frequency [Hz] :" ("Content"), w3500) -> (w3503:string)
                        n2466 = local read "EVENT LOG"() -> (w3505:string)
                        n2467 = call "Event Log.vi"("Content"=w3503, "EVENT LOG"=w3505) -> ("EVENT LOG"=w3504:string)  [unwired: 8 in, 1 out]
                        n2468 = local write "EVENT LOG"(w3504) -> ()
                      }
                      frame #22 {
                        n2469 = Wait (ms)(milliseconds to wait=u32 50) -> ()  [unwired: 1 out]
                      }
                      frame #23 {
                        n2470 = local read "NORMAL LOAD"() -> (w3508:dbl)
                        n2471 = Number To Fractional String(number=w3508, precision (6)=i16 2) -> (F-format string=w3509:string)  [unwired: 2 in]
                        n2472 = Concatenate Strings("Applied Load [grams] :" ("Content"), w3509) -> (w3511:string)
                        n2473 = local read "EVENT LOG"() -> (w3513:string)
                        n2474 = call "Event Log.vi"("Content"=w3511, "EVENT LOG"=w3513) -> ("EVENT LOG"=w3512:string)  [unwired: 8 in, 1 out]
                        n2475 = local write "EVENT LOG"(w3512) -> ()
                      }
                      frame #24 {
                        n2476 = Wait (ms)(milliseconds to wait=u32 50) -> ()  [unwired: 1 out]
                      }
                      frame #25 {
                        n2477 = local read "Set Strk"() -> (w3516:dbl)
                        n2478 = Number To Fractional String(number=w3516, precision (6)=i16 2) -> (F-format string=w3517:string)  [unwired: 2 in]
                        n2479 = Concatenate Strings("Set Stroke [mm] :" ("Content"), w3517) -> (w3519:string)
                        n2480 = local read "EVENT LOG"() -> (w3521:string)
                        n2481 = call "Event Log.vi"("Content"=w3519, "EVENT LOG"=w3521) -> ("EVENT LOG"=w3520:string)  [unwired: 8 in, 1 out]
                        n2482 = local write "EVENT LOG"(w3520) -> ()
                      }
                      frame #26 {
                        n2483 = Wait (ms)(milliseconds to wait=u32 50) -> ()  [unwired: 1 out]
                      }
                      frame #27 {
                        n2484 = local read "Set Temp"() -> (w3524:dbl)
                        n2485 = Number To Fractional String(number=w3524, precision (6)=i16 2) -> (F-format string=w3525:string)  [unwired: 2 in]
                        n2486 = Concatenate Strings("Set Temperature [deg C] :" ("Content"), w3525) -> (w3527:string)
                        n2487 = local read "EVENT LOG"() -> (w3529:string)
                        n2488 = call "Event Log.vi"("Content"=w3527, "EVENT LOG"=w3529) -> ("EVENT LOG"=w3528:string)  [unwired: 8 in, 1 out]
                        n2489 = local write "EVENT LOG"(w3528) -> ()
                      }
                      frame #28 {
                        n2490 = Wait (ms)(milliseconds to wait=u32 50) -> ()  [unwired: 1 out]
                      }
                      frame #29 {
                        n2491 = local read "Set Rh"() -> (w3532:dbl)
                        n2492 = Number To Fractional String(number=w3532, precision (6)=i16 2) -> (F-format string=w3533:string)  [unwired: 2 in]
                        n2493 = Concatenate Strings("Set Humidity [%RH] :" ("Content"), w3533) -> (w3535:string)
                        n2494 = local read "EVENT LOG"() -> (w3537:string)
                        n2495 = call "Event Log.vi"("Content"=w3535, "EVENT LOG"=w3537) -> ("EVENT LOG"=w3536:string)  [unwired: 8 in, 1 out]
                        n2496 = local write "EVENT LOG"(w3536) -> ()
                      }
                      frame #30 {
                        n2497 = Wait (ms)(milliseconds to wait=u32 50) -> ()  [unwired: 1 out]
                      }
                      frame #31 {
                        n2498 = local read "test time"() -> (w3540:dbl)
                        n2499 = Number To Fractional String(number=w3540, precision (6)=i16 1) -> (F-format string=w3541:string)  [unwired: 2 in]
                        n2500 = Concatenate Strings("Test Duration [mins] :" ("Content"), w3541) -> (w3543:string)
                        n2501 = local read "EVENT LOG"() -> (w3545:string)
                        n2502 = call "Event Log.vi"("Content"=w3543, "EVENT LOG"=w3545) -> ("EVENT LOG"=w3544:string)  [unwired: 8 in, 1 out]
                        n2503 = local write "EVENT LOG"(w3544) -> ()
                      }
                      frame #32 {
                        w3546 = dbl[] [] ("History Data")
                        w3547 = cluster{"y":dbl, dbl, "y":dbl}[] [] ("History Data")
                        w3548 = FALSE ("Visible")
                        n2504 = property on="Stroke ( mm )" class="WFChart (strict)"("History Data"=w3547) -> ()  [unwired: 2 in, 2 out]
                        n2505 = property on="Humidity ( %RH )" class="WFChart (strict)"("History Data"=w3546) -> ()  [unwired: 2 in, 2 out]
                        n2506 = property on="Temperature ( Deg C )" class="WFChart (strict)"("History Data"=w3546) -> ()  [unwired: 2 in, 2 out]
                        n2507 = property on="Electrical Contact Resistance ( % )" class="WFChart (strict)"("History Data"=w3546) -> ()  [unwired: 2 in, 2 out]
                        n2508 = property on="Coefficient of Friction" class="WFChart (strict)"("History Data"=w3546) -> ()  [unwired: 2 in, 2 out]
                        n2509 = property on="Frictional Force ( N )" class="WFChart (strict)"("History Data"=w3546) -> ()  [unwired: 2 in, 2 out]
                        n2510 = property on="Coefficient of Friction" class="WFChart (strict)"("History Data"=w3546) -> ()  [unwired: 2 in, 2 out]
                        n2511 = property on="Frictional Force ( N )" class="WFChart (strict)"("History Data"=w3546) -> ()  [unwired: 2 in, 2 out]
                        n2512 = property on="Electrical Contact Resistance ( % )" class="WFChart (strict)"("History Data"=w3546) -> ()  [unwired: 2 in, 2 out]
                        n2513 = property on="Humidity ( %RH )" class="WFChart (strict)"("History Data"=w3546) -> ()  [unwired: 2 in, 2 out]
                        n2514 = property on="Stroke ( mm )" class="WFChart (strict)"("History Data"=w3547) -> ()  [unwired: 2 in, 2 out]
                        n2515 = property on="Temperature ( Deg C )" class="WFChart (strict)"("History Data"=w3546) -> ()  [unwired: 2 in, 2 out]
                        n2516 = property on="Service Password Log" class="Str"("Visible"=w3548) -> ()  [unwired: 2 in, 2 out]
                        n2517 = property on="Password 3" class="Clust (strict)"("Visible"=w3548) -> ()  [unwired: 2 in, 2 out]
                      }
                    }
                    "TEST FILE NAM,E SAVED" <- TRUE ("TEST FILE NAM,E SAVED")
                  }
                }
              }
            }
          }
        }
        n2518 = case shown="True" w2845 {
          frame False {
            n2519 = local write "tfalg"(0.0 ("tfalg")) -> ()
          }
          frame True {
            n2520 = local read "tfalg"() -> (w2990:dbl)
            n2521 = Equal?(x=w2990, y=0.0) -> (x = y?=w2991:bool)
            n2522 = case shown="True" w2991 {
              frame False {
              }
              frame True {
                n2523 = local read "Total No. of Tests"() -> (w2994:dbl)
                n2524 = local write "tfalg"(1.0 ("tfalg")) -> ()
                n2525 = local write "acq 2"(FALSE ("acq 2")) -> ()
                n2526 = Wait (ms)(milliseconds to wait=u32 200) -> ()  [unwired: 1 out]
                n2527 = Increment(x=w2994) -> (x+1=w2993:dbl)
                n2528 = local write "Total No. of Tests"(w2993) -> ()
              }
            }
          }
        }
        n2529 = local write "Test \nStatus"(w2851) -> ()
        n2530 = local write "Save"(w2851) -> ()
        n2531 = local read "Main Tab"() -> (w2808:T2)
        n2532 = case shown="True" w2832 {
          tunnel: [FALSE ("RUN") TRUE ("RUN")] -> w2831
          tunnel: [_ 1] -> w2824
          frame False {
          }
          frame True {
          }
        }
        n2533 = In Range and Coerce(upper limit=w2839, x=w2812, lower limit=w2838) -> (In Range?=w2830:bool)  [unwired: 1 out]
        n2534 = In Range and Coerce(upper limit=w2836, x=w2811, lower limit=w2837) -> (In Range?=w2828:bool)  [unwired: 1 out]
        n2535 = case shown="True" w2844 {
          frame False {
            n2536 = local read "Rt 3"() -> (w2972:bool)
            n2537 = case shown="True" w2972 {
              frame False {
              }
              frame True {
                n2538 = local write "Rt 3"(FALSE ("Rt 3")) -> ()
                n2539 = local write "Json End Flg"(TRUE ("Upld AR 2")) -> ()
              }
            }
            "Rt" <- TRUE ("Rt")
            "Rt 2" <- FALSE ("Rt")
          }
          frame True {
            n2540 = local read "Rt"() -> (w2979:bool)
            n2541 = local write "Rt 2"(TRUE ("Rt 2")) -> ()
            n2542 = case shown="True" w2979 {
              frame False {
              }
              frame True {
                w2980 = TRUE ("Upld AR 2")
                n2543 = local write "Rt"(FALSE ("Rt")) -> ()
                n2544 = local write "Upld AR"(w2980) -> ()
                n2545 = local write "Json St Flg"(w2980) -> ()
              }
            }
            "Rt 3" <- TRUE ("Rt 3")
          }
        }
        n2546 = case shown="True" w2830 {
          tunnel: [FALSE ("RUN") TRUE ("RUN")] -> w2829
          tunnel: [_ 2] -> w2823
          frame False {
          }
          frame True {
          }
        }
        n2547 = case shown="True" w2828 {
          tunnel: [FALSE ("RUN") TRUE ("RUN")] -> w2827
          tunnel: [_ 3] -> w2822
          frame False {
          }
          frame True {
          }
        }
        n2548 = case shown="\"Acquire\"" w2808 {
          tunnel: w2810 -> [_ w3041]
          frame Default {
            w3040 = 0.0 ("output")
            n2549 = local write "PID-out"(w3040) -> ()
            n2550 = local write "Frequency ( Hz )"(w3040) -> ()
          }
          frame "Acquire" {
            n2551 = stacked-sequence {
              frame #0 {
                n2552 = local read "Auto Start Test"() -> (w3043:bool)
                n2553 = case shown="True" w3043 {
                  tunnel: "RUN" -> [w3064 w3067]
                  tunnel: [w3064 w3066] -> w3044
                  frame False {
                  }
                  frame True {
                    n2554 = local read "Auto Start Temp"() -> (w3065:bool)
                    n2555 = Or(x=w3067, y=w3065) -> (x .or. y?=w3066:bool)
                  }
                }
                n2556 = local read "clk"() -> (w3063:dbl)
                n2557 = local read "Save"() -> (w3059:bool)
                n2558 = Equal?(x=w3063, y=0.0) -> (x = y?=w3060:bool)
                n2559 = And(x=w3060, y=w3059) -> (x .and. y?=w3061:bool)
                n2560 = Not(x="Engage") -> (.not. x?=w3050:bool)
                n2561 = case shown="False" w3044 {
                  tunnel: [0.0 w3090] -> w3046
                  frame False {
                    (unwired) TRUE ("Visible")
                    n2562 = local read "Auto Start Test"() -> (w3071:bool)
                    n2563 = local write "Start Time"(TRUE ("Start Time")) -> ()
                    n2564 = property on="Stroke 2" class="DigNum (strict)"("Visible"=FALSE) -> ()  [unwired: 2 in, 2 out]
                    n2565 = case shown="False" w3071 {
                      frame False {
                        n2566 = property on="Heater Button" class="Bool (strict)"("DisabledEnum"=T17."Enabled" ("Disabled")) -> ()  [unwired: 2 in, 2 out]
                        n2567 = property on="Humidity" class="Bool (strict)"("DisabledEnum"=T17."Enabled" ("Disabled")) -> ()  [unwired: 2 in, 2 out]
                      }
                      frame True {
                      }
                    }
                    n2568 = case shown="False" "TestCompFlg" {
                      frame False {
                        n2569 = local read "StartFlg"() -> (w3079:bool)
                        n2570 = case shown="True" w3079 {
                          frame False {
                          }
                          frame True {
                            n2571 = stacked-sequence {
                              frame #0 {
                                n2572 = local read "EVENT LOG"() -> (w3083:string)
                                n2573 = call "Event Log.vi"("Content"="Test was interrupted", "EVENT LOG"=w3083) -> ("EVENT LOG"=w3084:string)  [unwired: 8 in, 1 out]
                                n2574 = local write "EVENT LOG"(w3084) -> ()
                                n2575 = property on="RUN" class="Bool (strict)"("Visible"=TRUE) -> ()  [unwired: 2 in, 2 out]
                                n2576 = property on="Auto Start Test" class="Bool (strict)"("Visible"=TRUE) -> ()  [unwired: 2 in, 2 out]
                              }
                              frame #1 {
                                w3086 = FALSE ("StartFlg")
                                n2577 = property on="Heater Button" class="Bool (strict)"("Val(Sgnl)"=FALSE ("Value (Signaling)")) -> ()  [unwired: 2 in, 2 out]
                                n2578 = local write "Heater Button"(w3086) -> ()
                                n2579 = local write "StartFlg"(w3086) -> ()
                                n2580 = local write "Humidity"(w3086) -> ()
                              }
                              frame #2 {
                                n2581 = local write "Command"("VC;0" ("Command")) -> ()
